vi "Do.vi"(6 "Input":variant, 8 "error in":errorcluster, 9 "Self Enqueuer":refnum<class "Message Enqueuer.lvclass">, 10 "Series Enqueuer":refnum<class "Message Enqueuer.lvclass">, 11 "Sample PWM Fan in":refnum<class "Sample PWM Fan.lvclass">) -> (0 "error out":errorcluster, 3 "Sample PWM Fan out":refnum<class "Sample PWM Fan.lvclass">)   [LabVIEW 2023, in "Sample PWM Fan.lvclass"]
uses:
  Sample PWM Fan.lvclass
  <vilib>/ActorFramework/Message Enqueuer/Message Enqueuer.lvclass
  Task/Task Base/Task Base.lvclass/Task Base.ctl
  Series/ISeries Actor/ISeries Actor Messages/Point Data Updated Msg/Point Data Updated Msg.lvclass/Point Data Updated Msg.ctl
  <vilib>/ActorFramework/Message Enqueuer/Message Enqueuer.lvclass/Message Enqueuer.ctl
  <vilib>/ActorFramework/Message Enqueuer/Enqueue.vi
  Series/ISeries Actor/ISeries Actor Messages/Point Data Updated Msg/Point Data Updated Msg.lvclass
  <vilib>/Utility/LVClass/Get LV Class Name.vi
  <resource>/AFDebug/Generate Trace for Message.vi
  <vilib>/ActorFramework/Message Priority Queue/Priority Enqueue.vi
  Task/Task Base/Task Base.lvclass
  Measure and Stimulus Subsystems/Measure and Stimulus Subsystems.lvclass
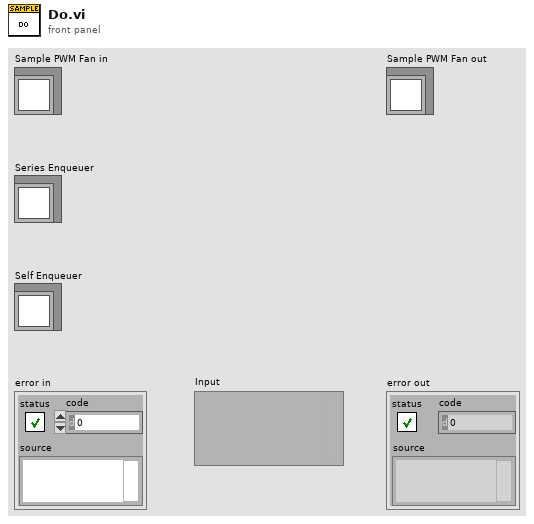
[diagram p1: front panel]
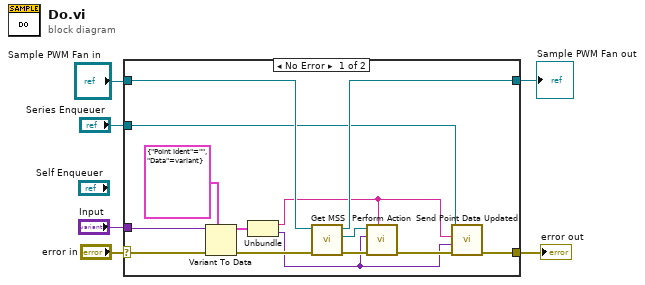
[diagram p0: block diagram]
diagram:
  n1 = case shown="No Error" "error in" {
    selector: "error in" -> [w16 w22]
    tunnel: [w8 w22] -> w5
    tunnel: [w17 w21] -> w3
    tunnel: "Sample PWM Fan in" -> [w20 w21]
    tunnel: "Input" -> [w13 _]
    tunnel: "Series Enqueuer" -> [w11 _]
    frame No Error {
      n2 = Variant To Data(error in=w16, type=cluster{"Point Ident":string, "Data":variant} {"Point Ident"="", "Data"=variant}, Variant=w13) -> (data=w12:cluster{"Point Ident":string, "Data":variant}, error out=w15:errorcluster)
      n3 = Unbundle(w12) -> ("Point Ident"=w10:string, "Data"=w7:variant)
      n4 = call "Get MSS.vi"("error in (no error)"=w15, "Task Base in"=w20) -> ("error out"=w18:errorcluster, "MSS"=w19:refnum<class "Measure and Stimulus Subsystems.lvclass">, "Task Base out"=w17:refnum<class "Sample PWM Fan.lvclass">)  [unwired: 7 in]
      n5 = call "Perform Action.vi"("Point Ident"=w10, "error in"=w18, "Input"=w7, "MSS in"=w19) -> ("error out"=w9:errorcluster)  [unwired: 5 in, 2 out]
      n6 = call "Send Point Data Updated.vi"("error in (no error)"=w9, "Data"=w7, "Point Ident"=w10, "Message Enqueuer"=w11) -> ("error out"=w8:errorcluster)  [unwired: 6 in, 1 out]
    }
    frame Error {
    }
  }
  "error out" <- w5
  "Sample PWM Fan out" <- w3
